vi "toXml.vi"(8 "error in (no error)":errorcluster, 11 "Channel in":refnum<class "Channel.lvclass">) -> (0 "error out":errorcluster, 2 "xmlNode":refnum<class "xmlNode.lvclass">, 3 "Channel out":refnum<class "Channel.lvclass">)   [LabVIEW 2011, in "Tools.lvlib" / "DatabaseHelpers.lvlib" / "Channel.lvclass"]
uses:
  Channel.lvclass
  xmlNode/xmlNode.lvclass
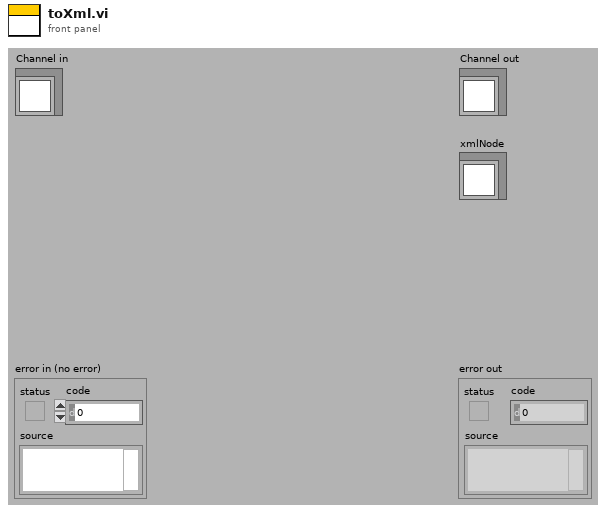
[diagram p1: front panel]
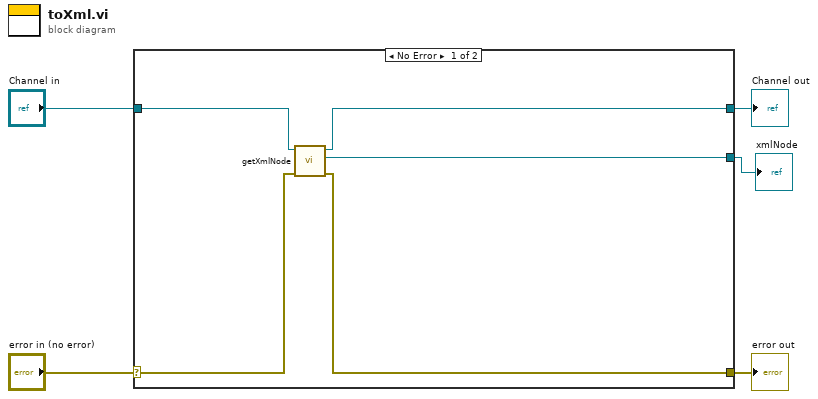
[diagram p0: block diagram]
diagram:
  n1 = case shown="No Error" "error in (no error)" {
    selector: "error in (no error)" -> [w7 w12]
    tunnel: [w6 w12] -> w4
    tunnel: [w9 w11] -> w2
    tunnel: "Channel in" -> [w10 w11]
    tunnel: [w8 _] -> w1
    frame No Error {
      n2 = call "getXmlNode.vi"("error in (no error)"=w7, "Channel.lvclass in"=w10) -> ("error out"=w6:errorcluster, "xmlNode"=w8:refnum<class "xmlNode.lvclass">, "Channel.lvclass out"=w9:refnum<class "Channel.lvclass">)  [unwired: 7 in]
    }
    frame Error {
    }
  }
  "error out" <- w4
  "Channel out" <- w2
  "xmlNode" <- w1
